vi "set_y_amplitude.vi"(8 "error in (no error)":errorcluster, 10 "y amplitude":dbl[unit], 11 "TrajectoryTS090820Circular2D in":refnum<class "TrajectoryTS090820Circular2D.lvclass">) -> (0 "error out":errorcluster, 3 "TrajectoryTS090820Circular2D out":refnum<class "TrajectoryTS090820Circular2D.lvclass">)   [LabVIEW 2010, in "TrajectoryTS090820Circular2D.lvclass"]
uses:
  TrajectoryTS090820Circular2D.lvclass
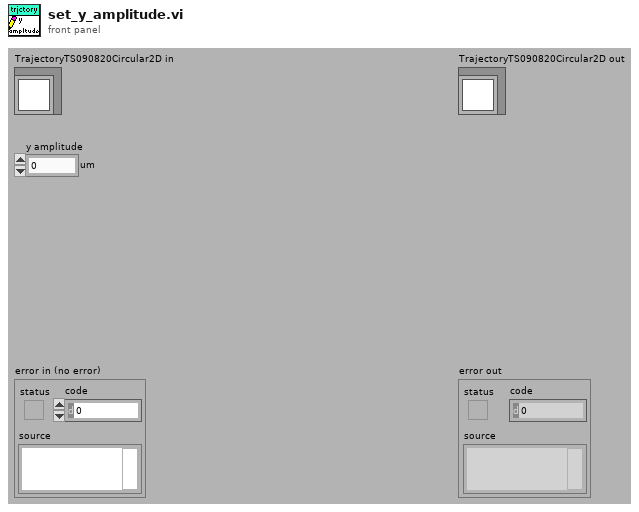
[diagram p1: front panel]
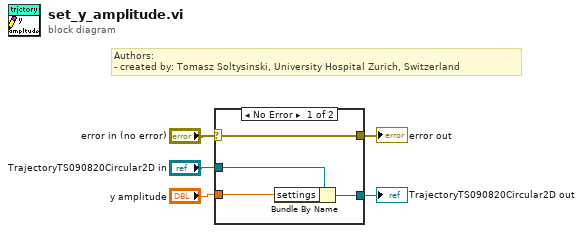
[diagram p0: block diagram]
diagram:
  # "Authors: \n- created by: Tomasz Soltysinski, University Hospital Zurich, Switzerland"
  n1 = case shown="No Error" "error in (no error)" {
    selector: "error in (no error)" -> [w6 w10]
    tunnel: [w6 w10] -> w4
    tunnel: [w8 w11] -> w2
    tunnel: "TrajectoryTS090820Circular2D in" -> [w9 w11]
    tunnel: "y amplitude" -> [w7 _]
    frame No Error {
      n2 = Bundle By Name(cluster=w9, "settings"=w7) -> (w8:refnum<class "TrajectoryTS090820Circular2D.lvclass">)
    }
    frame Error {
    }
  }
  "error out" <- w4
  "TrajectoryTS090820Circular2D out" <- w2
